vi "Rings on the left.vi"(0 "Iteration":i32, 5 "Revolution (steps)":i32, 7 "Separation (angle)":i32, 9 "Change colours?":bool) -> ()   [LabVIEW 2017]
doc: "To draw rings on the left side of the round object and move to the right side once left side is finished drawing.\n\n<b>P.s.</b> Left right for horizontal view and top bottom for vertical view."
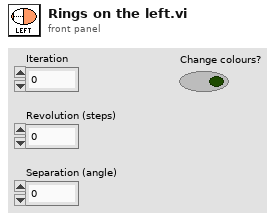
[diagram p1: front panel]
types:
  T1 = enum16{"Full", "Half", "Quarter", "Eighth", "Sixteenth"}
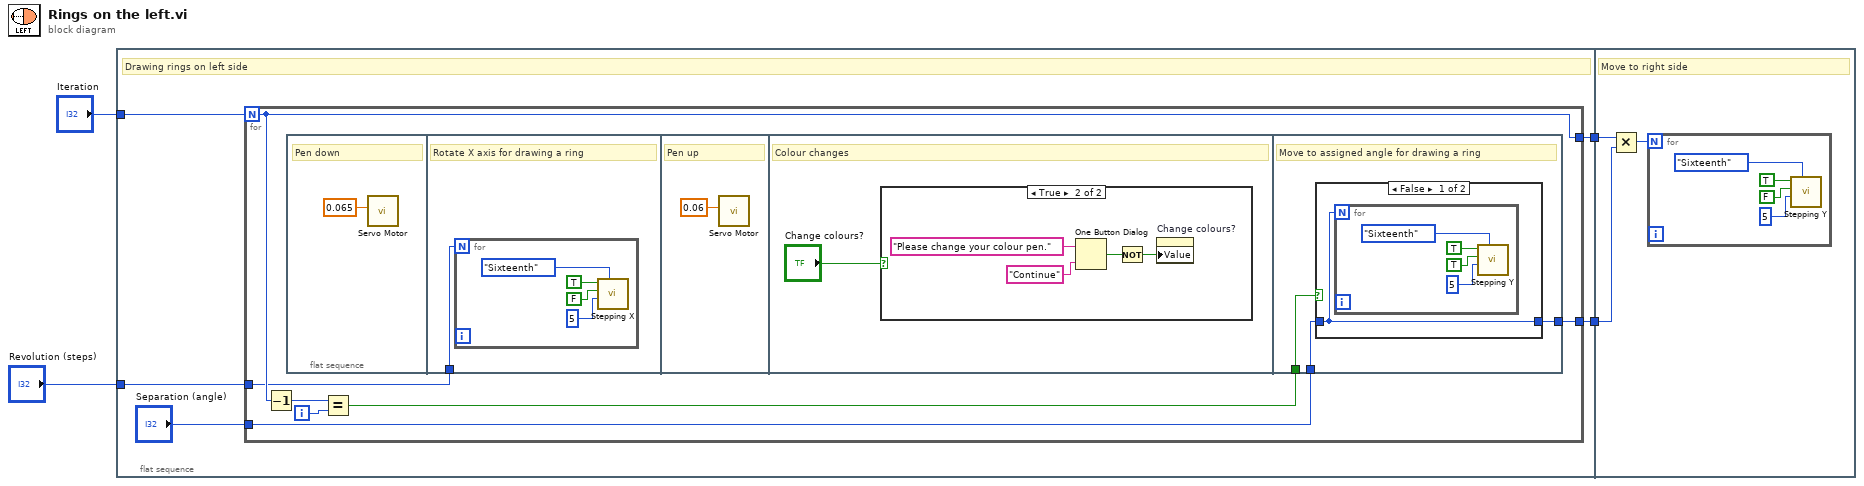
[diagram p0: block diagram]
diagram:
  n1 = flat-sequence {
    tunnel: [w9] -> w4
    tunnel: [w8] -> w3
    tunnel: "Iteration" -> [w7]
    tunnel: "Revolution (steps)" -> [w6]
    tunnel: w4 -> [w39]
    tunnel: w3 -> [w38]
    frame #0 {
      # "Drawing rings on left side"
      n2 = for {
        N: w7 -> [w13]
        tunnel: [w13] -> w9
        tunnel: [w12] -> w8
        tunnel: w6 -> [w11]
        tunnel: "Separation (angle)" -> [w10]
        i -> [w15]
        n3 = Decrement(x=w13) -> (x-1=w16:i32)
        n4 = flat-sequence {
          tunnel: w11 -> [w18]
          tunnel: w14 -> [w31]
          tunnel: [w30] -> w12
          tunnel: w10 -> [w29]
          frame #0 {
            # "Pen down"
            n5 = call "Servo Motor.vi"("Duty Cycle"=0.065) -> ()  [unwired: 9 in, 2 out]
          }
          frame #1 {
            # "Rotate X axis for drawing a ring"
            n6 = for {
              N: w18 -> [_]
              n7 = call "Stepping X.vi"("Microstep size"=T1."Sixteenth", "Speed"=u32 5, "Direction"=FALSE, "Enable"=TRUE) -> ()  [unwired: 7 in, 1 out]
            }
          }
          frame #2 {
            # "Pen up"
            n8 = call "Servo Motor.vi"("Duty Cycle"=0.06) -> ()  [unwired: 9 in, 2 out]
          }
          frame #3 {
            # "Colour changes"
            n9 = case shown="True" "Change colours?" {
              frame False {
              }
              frame True {
                n10 = One Button Dialog(message="Please change your colour pen.", button name ("OK")="Continue") -> (true=w27:bool)
                n11 = Not(x=w27) -> (.not. x?=w28:bool)
                n12 = property on="Change colours?" class="Bool (strict)"("Value"=w28) -> ()  [unwired: 2 in, 2 out]
              }
            }
          }
          frame #4 {
            # "Move to assigned angle for drawing a ring"
            n13 = case shown="False" w31 {
              tunnel: [w32 w37] -> w30
              tunnel: w29 -> [w32 w37]
              frame False {
                n14 = for {
                  N: w32 -> [_]
                  n15 = call "Stepping Y.vi"("Microstep size"=T1."Sixteenth", "Speed"=u32 5, "Direction"=TRUE, "Enable"=TRUE) -> ()  [unwired: 7 in, 1 out]
                }
              }
              frame True {
              }
            }
          }
        }
        n16 = Equal?(x=w16, y=w15) -> (x = y?=w14:bool)
      }
    }
    frame #1 {
      # "Move to right side"
      n17 = Multiply(x=w39, y=w38) -> (x*y=w40:i32)
      n18 = for {
        N: w40 -> [_]
        n19 = call "Stepping Y.vi"("Microstep size"=T1."Sixteenth", "Speed"=u32 5, "Direction"=FALSE, "Enable"=TRUE) -> ()  [unwired: 7 in, 1 out]
      }
    }
  }
